vi "ProcessChromaloxMessage.vi"(5 "Chromalox Message":string, 9 "error in (no error)":errorcluster) -> (6 "Array 3":string[](array[string]), 8 "Reading":dbl, 10 "Units":string, 15 "error out":errorcluster)   [LabVIEW 2017, in "Thermal Shock.lvlib"]
uses:
  Thermal Shock.lvlib
panel:
  out "Uncasted hex":string
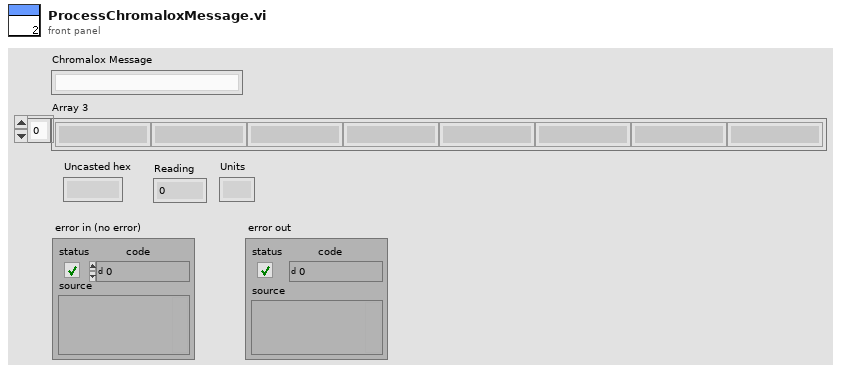
[diagram p1: front panel]
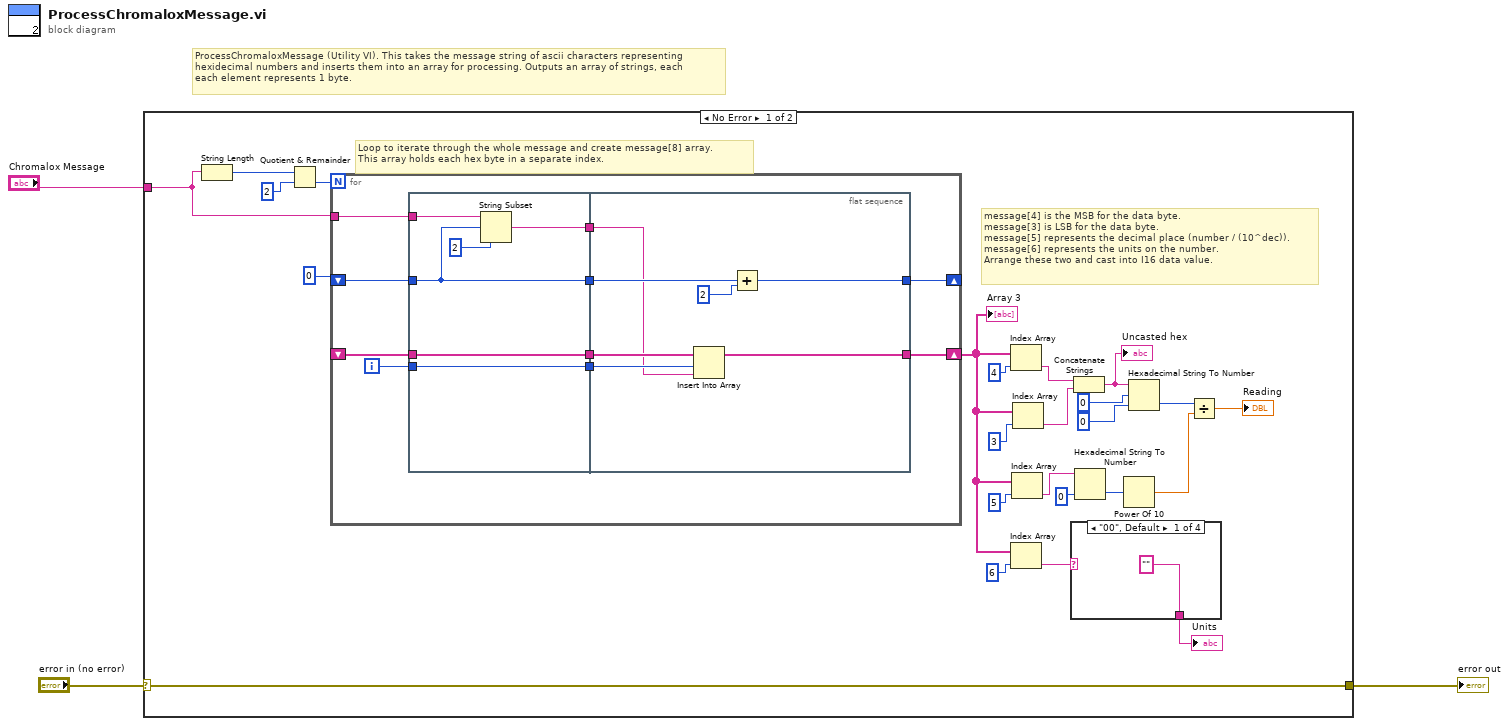
[diagram p0: block diagram]
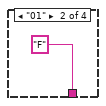
[diagram p2: hidden frame]
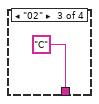
[diagram p3: hidden frame]
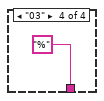
[diagram p4: hidden frame]
diagram:
  # "ProcessChromaloxMessage (Utility VI). This takes the message string of ascii characters representing \nhexidecimal numbers and inserts them into an array for processing. Outputs an array of strings, each\neach element represents 1 byte."
  n1 = case shown="No Error" "error in (no error)" {
    selector: "error in (no error)" -> [w26 w55]
    tunnel: "Chromalox Message" -> [w27 _]
    tunnel: [w26 w55] -> w1
    frame No Error {
      # "message[4] is the MSB for the data byte. \nmessage[3] is LSB for the data byte.\nmessage[5] represents the decimal place (number / (10^dec)).\nmessage[6] represents the units on the number.\nArrange these two and cast into I16 data value."
      # "Loop to iterate through the whole message and create message[8] array.\nThis array holds each hex byte in a separate index."
      n2 = String Length(string=w27) -> (length=w17:i32)
      n3 = Quotient & Remainder(x=w17, y=2) -> (floor(x/y)=w22:i32)  [unwired: 1 out]
      n4 = for {
        N: w22 -> [_]
        tunnel: w27 -> [w41]
        shift-right: [w38] -> _
        shift-left: 0 -> [w40]
        shift-right: [w32] -> w11
        shift-left: _ -> [w34]
        i -> [w36]
        n5 = flat-sequence {
          tunnel: w41 -> [w47]
          tunnel: w40 -> [w45]
          tunnel: [w45] -> w39
          tunnel: [w44] -> w37
          tunnel: w36 -> [w43]
          tunnel: [w43] -> w35
          tunnel: w34 -> [w42]
          tunnel: [w42] -> w33
          tunnel: w39 -> [w54]
          tunnel: [w53] -> w38
          tunnel: w37 -> [w48]
          tunnel: w35 -> [w49]
          tunnel: w33 -> [w51]
          tunnel: [w50] -> w32
          frame #0 {
            n6 = String Subset(string=w47, offset (0)=w45, length (rest)=2) -> (substring=w44:string)
          }
          frame #1 {
            n7 = Insert Into Array(array=w51, index=w49, new element=w48) -> (w50:string[])
            n8 = Add(x=w54, y=2) -> (x+y=w53:i32)
          }
        }
      }
      "Array 3" <- w11
      n9 = Index Array(array=w11, index=4) -> (element=w20:string)
      n10 = Index Array(array=w11, index=6) -> (element=w13:string)
      n11 = Index Array(array=w11, index=5) -> (element=w9:string)
      n12 = Index Array(array=w11, index=3) -> (element=w19:string)
      n13 = case shown="\"00\", Default" w13 {
        tunnel: ["" "F" "C" "%"] -> w12
        frame "00", Default {
        }
        frame "01" {
        }
        frame "02" {
        }
        frame "03" {
        }
      }
      "Units" <- w12
      n14 = Concatenate Strings(w20, w19) -> (w16:string)
      "Uncasted hex" <- w16
      n15 = Hexadecimal String To Number(string=w9, default (0uL)=i16 0 ("default (0 U32)")) -> (number=w5:i16)  [unwired: 1 in, 1 out]
      n16 = Power Of 10(x=w5) -> (10^x=w4:dbl)
      n17 = Hexadecimal String To Number(string=w16, offset=0, default (0uL)=i16 0 ("default (0 U32)")) -> (number=w7:i16)  [unwired: 1 out]
      n18 = Divide(x=w7, y=w4) -> (x/y=→"Reading":dbl)
    }
    frame Error {
    }
  }
  "error out" <- w1
